vi "Process Block Diagram.vi"(8 "error in (no error)":errorcluster, 11 "vi ref":refnum<vi>) -> (0 "error out":errorcluster, 1 "sub vi loc":T1[](array[typedef]), 2 "sub vi refs":refnum<vi>[](array[refnum]))   [LabVIEW 2014, in "lvprj2html.lvlib"]
uses:
  lvprj2html.lvlib
  <vilib>/Utility/miscctls.llb/LVRectTypeDef.ctl
  <vilib>/Utility/traverseref.llb/TRef TravTarget.ctl
  <vilib>/Utility/traverseref.llb/VI Scripting - Traverse.lvlib
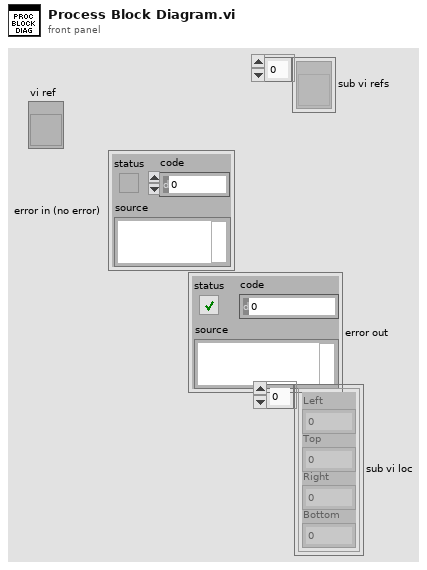
[diagram p1: front panel]
types:
  T1 = typedef "LVRectTypeDef.ctl" = cluster{"Left":i16, "Top":i16, "Right":i16, "Bottom":i16}
  T2 = typedef "TRef TravTarget.ctl" = enum16{"FP", "BD", "Other"}
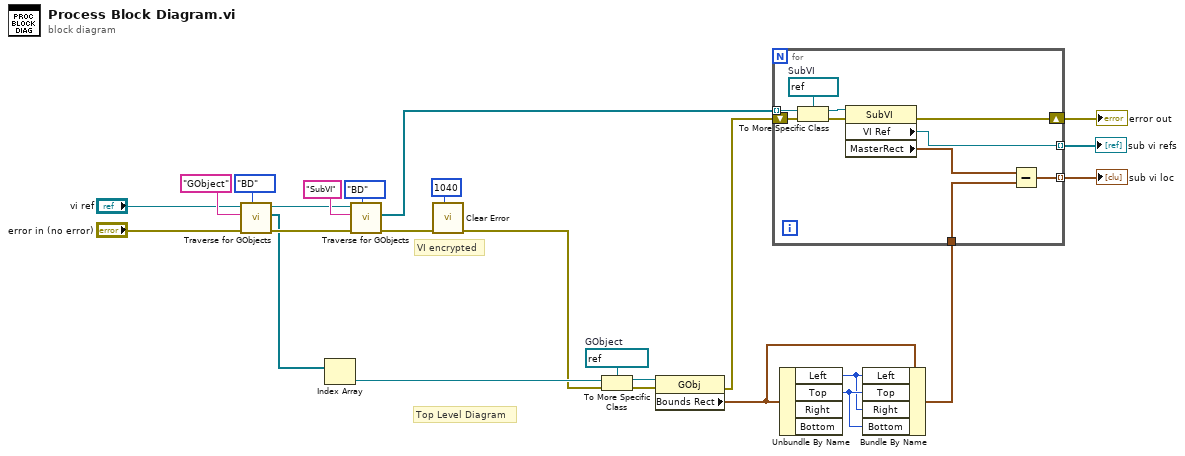
[diagram p0: block diagram]
diagram:
  w13 = refnum<vi> refnum  # GObject
  # "Top Level Diagram"
  # "VI encrypted"
  n1 = call <vilib>:"Traverse for GObjects.vi"("Traverse Target"=TRef_TravTarget."BD", "error in (no error)"="error in (no error)", "Class Name"="GObject", "VI Refnum"="vi ref") -> ("error out"=w17:errorcluster, "References"=w15:refnum<vi>[], "dup VI Refnum"=w18:refnum<vi>)  [unwired: 4 in, 1 out]
  n2 = Index Array(array=w15) -> (element=w12:refnum<vi>)  [unwired: 1 in]
  n3 = call <vilib>:"Traverse for GObjects.vi"("Traverse Target"=TRef_TravTarget."BD", "error in (no error)"=w17, "Class Name"="SubVI", "VI Refnum"=w18) -> ("error out"=w23:errorcluster, "References"=w25:refnum<vi>[])  [unwired: 4 in, 2 out]
  n4 = call "Clear Error.vi"("code"=1040, "error in (no error)"=w23) -> ("error out"=w2:errorcluster)  [unwired: 8 in, 1 out]
  n5 = To More Specific Class(target class=w13, reference=w12, error in=w2) -> (specific class reference=w14:refnum<vi>, error out=w5:errorcluster)
  n6 = property class="GObj"(reference=w14, error in=w5) -> (error out=w4:errorcluster, "Bounds Rect"=w9:T1)  [unwired: 1 out]
  n7 = Unbundle By Name(w9) -> ("Left"=w10:i16, "Top"=w11:i16)  [unwired: 2 out]
  n8 = Bundle By Name(cluster=w9, "Left"=w10, "Top"=w11, "Right"=w10, "Bottom"=w11) -> (w8:T1)
  n9 = for {
    tunnel: w25 -> [w34] mode=indexing
    tunnel: [w31] -> w16 mode=indexing
    tunnel: w8 -> [w30]
    shift-right: [w26] -> w3
    shift-left: w4 -> [w29]
    tunnel: [w27] -> w1 mode=indexing
    w35 = refnum<vi> refnum  # SubVI
    n10 = To More Specific Class(target class=w35, reference=w34, error in=w29) -> (specific class reference=w33:refnum<vi>, error out=w28:errorcluster)
    n11 = property class="SubVI"(reference=w33, error in=w28) -> (error out=w26:errorcluster, "VI Ref"=w27:refnum<vi>, "MasterRect"=w32:T1)  [unwired: 1 out]
    n12 = Subtract(x=w32, y=w30) -> (x-y=w31:T1)
  }
  "error out" <- w3
  "sub vi loc" <- w16
  "sub vi refs" <- w1
